vi "Overlay detection problem.vi"(0 "Font, Size & Style":T2, 1 "Font Size":dbl, 2 "Image In":T1, 3 "Origin":cluster{"X Target":sgl, dbl}, 4 "Detection string":string) -> (5 "Image Out":T1)   [LabVIEW 2013]
uses:
  <vilib>/vision/Image Controls.llb/IMAQ Image.ctl
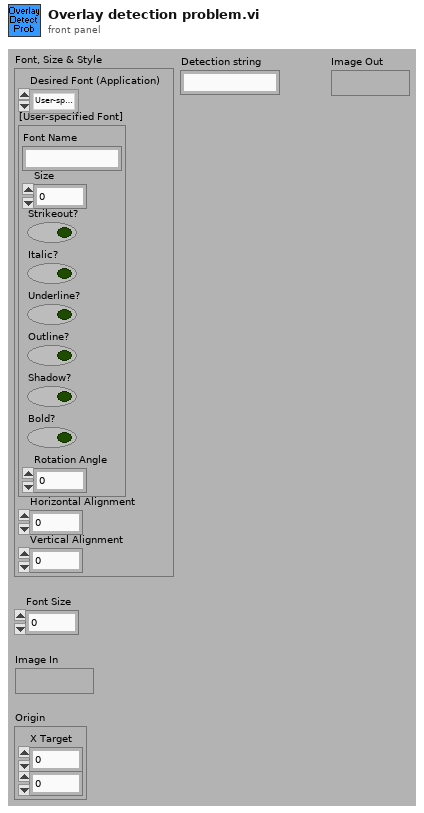
[diagram p1: front panel]
types:
  T1 = typedef "IMAQ Image.ctl" = refnum<image>
  T2 = cluster{"Desired Font (Application)":enum16{"User-specified Font", "Application Font", "System Font", "Dialog Font"}, "[User-specified Font]":cluster{"Font Name":string, "Size":i16, "Strikeout?":bool, "Italic?":bool, "Underline?":bool, "Outline?":bool, "Shadow?":bool, "Bold?":bool, "Rotation Angle":dbl}, "Horizontal Alignment":i16, "Vertical Alignment":i16}
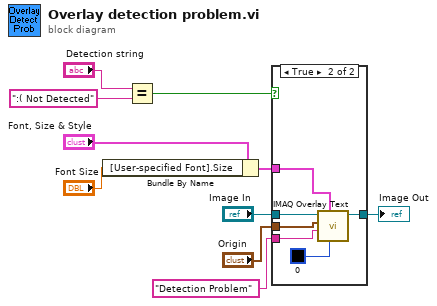
[diagram p0: block diagram]
diagram:
  n1 = Bundle By Name(cluster="Font, Size & Style", "[User-specified Font].Size"="Font Size") -> (w8:T2)
  n2 = Equal?(x="Detection string", y=":( Not Detected") -> (x = y?=w2:bool)
  n3 = case shown="True" w2 {
    tunnel: "Image In" -> [w11 w17]
    tunnel: [w11 w16] -> w10
    tunnel: "Detection Problem" ("String") -> [_ w15]
    tunnel: "Origin" -> [_ w14]
    tunnel: w8 -> [_ w13]
    frame False {
    }
    frame True {
      n4 = call "IMAQ Overlay Text"("Text Color (black)"=u32 0 ("Color"), "Font, Size & Style"=w13, "String"=w15, "Origin"=w14, "Image"=w17) -> ("Image Out"=w16:T1)  [unwired: 5 in, 1 out]
    }
  }
  "Image Out" <- w10
